vi "helloworld.vi"(11 "Inputs":string[](array[string])) -> (2 "Output/Failure":string, 3 "CLI Process Return Code":i32)   [LabVIEW 2017]
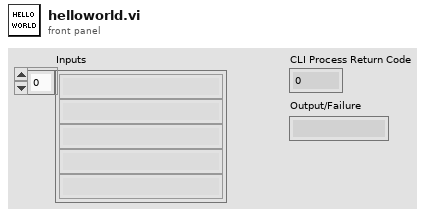
[diagram p1: front panel]
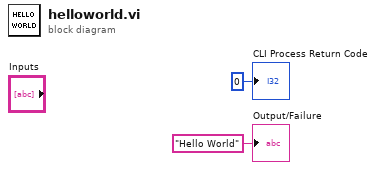
[diagram p0: block diagram]
diagram:
  "Output/Failure" <- "Hello World" ("Output")
  "CLI Process Return Code" <- 0 ("CLI Process Return Code")
